vi "ZK Create MB.vi"() -> ()   [LabVIEW 2016, in "质控单元V4.lvlib"]
uses:
  <vilib>/Plasmionique/MB Master/MB_Master_Serial/MB_Master_Serial.lvclass
  C:/Program Files (x86)/National Instruments/LabVIEW 2016/vi.lib/Plasmionique/MB Master/MB_Master/MB_Master.lvclass
  <vilib>/Plasmionique/MB Master/MB_Master_TCP/MB_Master_TCP.lvclass
  <vilib>/Plasmionique/MB Master/MB_Master/MB_Master.lvclass
panel:
  out "auto connected":bool=TRUE
  out "error out":errorcluster
  out "Connected":bool
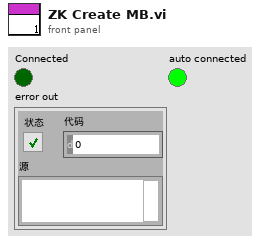
[diagram p1: front panel]
types:
  T1 = cluster{"baud rate (bps)":u32, "stop bits":u16, "parity":u16, "flow control":u16, "timeout":u32, "retries":i32}
  T2 = typedef "质控单元V4.lvlib/质控slave id.ctl" = enum16{"null", "氨氮", "总磷", "总氮", "CODMn", "CODCr"}
  T3 = cluster{"氨氮":bool, "总磷":bool, "总氮":bool, "CODMn":bool, "CODCr":bool, "氨氮总磷":bool, "总磷总氮":bool}
  T4 = typedef "质控单元V4.lvlib/质控仪器状态显示.ctl" = cluster{"运行模式":string, "运行状态":string, "液位状态":string, "告警状态":string, "当前流程":string, "当前步骤":string, "剩余时间":string}
  T5 = typedef "质控单元V4.lvlib/质控仪器状态.ctl" = cluster{"运行状态":enum16{"待机", "润洗", "进样", "定量", "加标", "等待取样", "排液", "异常停机"}, "液位状态":enum16{"无感应", "有感应"}, "告警状态":enum16{"无告警", "液位故障告警", "注射泵异常"}, "当前步骤数":u16, "当前步骤剩余时间":u16, "当前步骤具体操作":enum16{"加标", "进样", "排液", "搅拌", "定量"}, "当前流程":enum16{"待机", "进样流程", "加标流程", "排液流程", "水样润洗流程", "加标润洗流程"}}
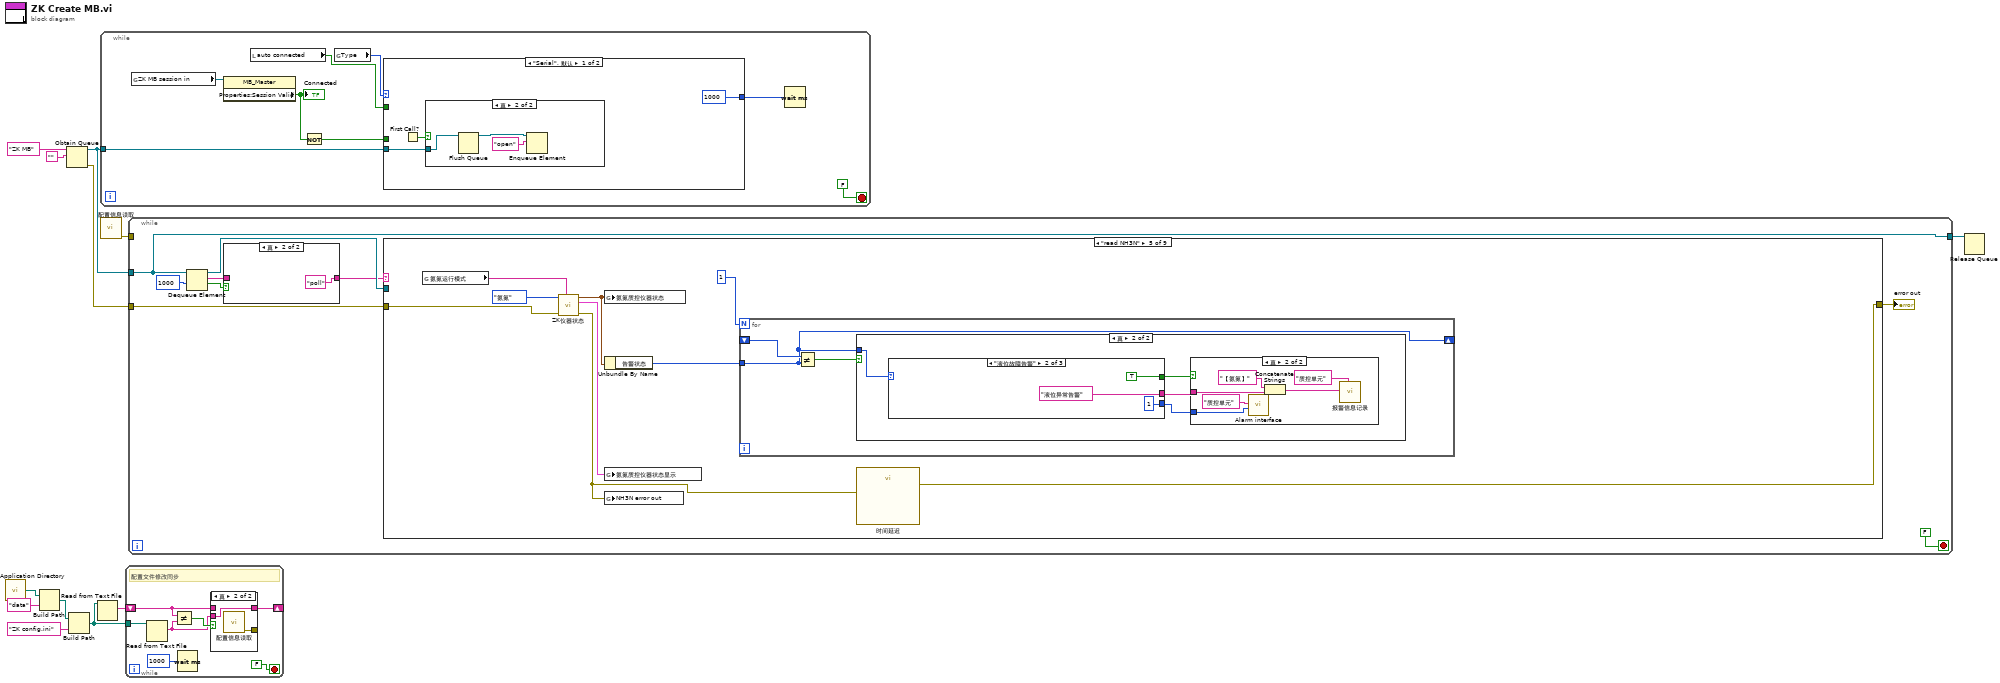
[diagram p0: block diagram]
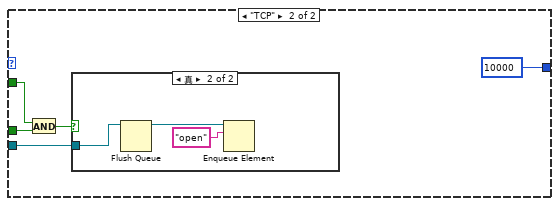
[diagram p4: hidden frame]
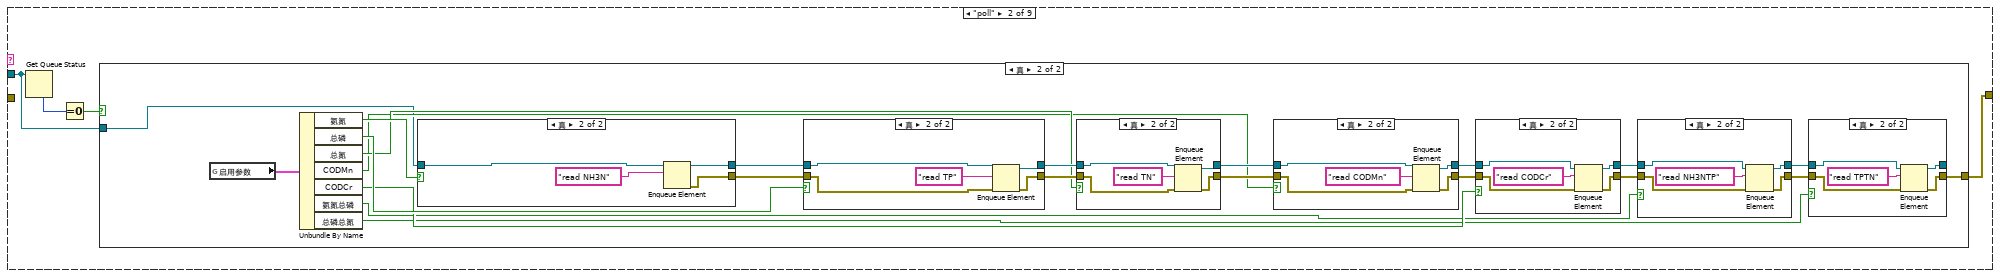
[diagram p8: hidden frame]
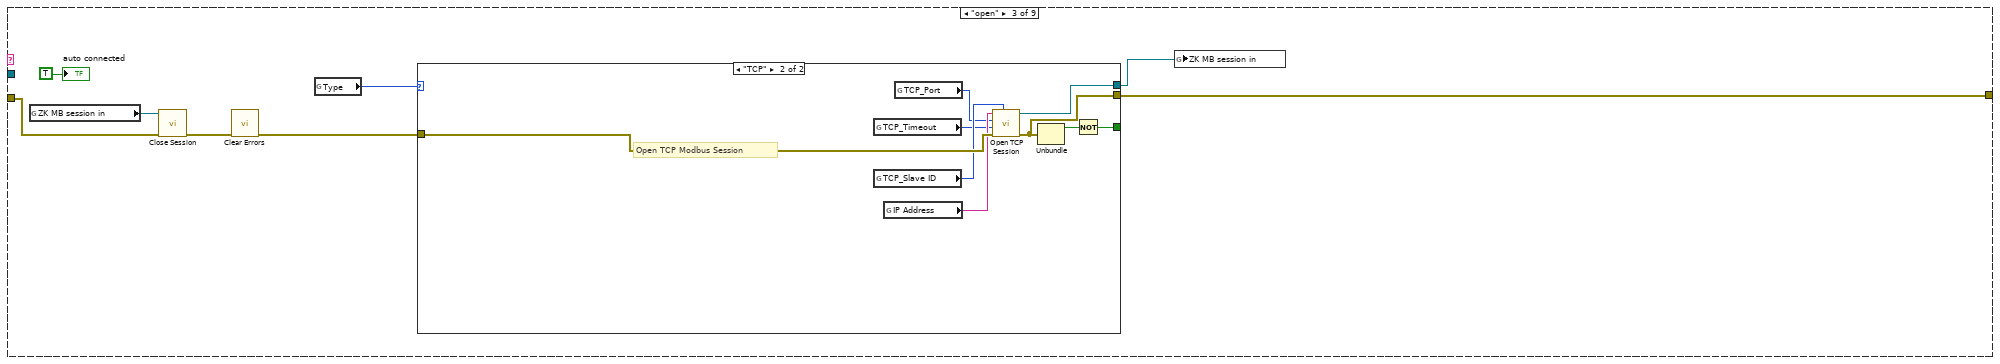
[diagram p17: hidden frame]
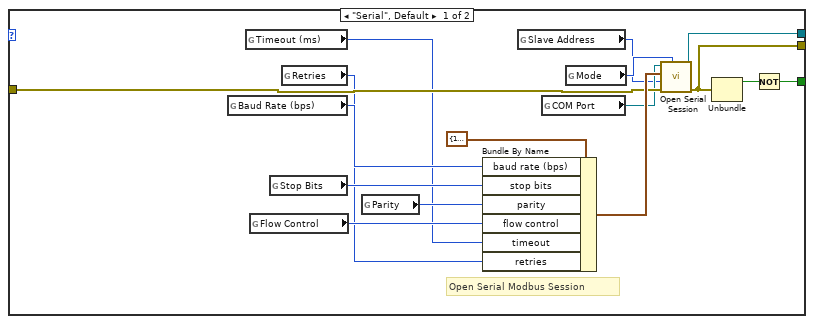
[diagram p18: hidden frame]
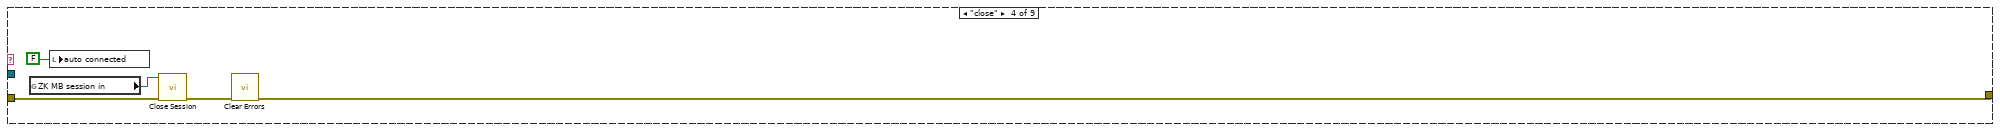
[diagram p19: hidden frame]
diagram:
  n1 = call <vilib>:"Application Directory.vi"() -> ("Application Directory"=w6:path)
  n2 = Build Path(base path=w6, name or relative path="data" ("名称或相对路径")) -> (appended path=w3:path)
  n3 = Obtain Queue(name (unnamed)="ZK MB" ("名称（未命名）"), element data type="") -> (queue out=w10:refnum<queue>, error out=w8:errorcluster)  [unwired: 3 in, 1 out]
  n4 = Build Path(base path=w3, name or relative path="ZK config.ini" ("名称或相对路径")) -> (appended path=w1:path)
  n5 = Read from Text File(file (use dialog)=w1) -> (text=w2:string)  [unwired: 3 in, 3 out]
  n6 = while {
    tunnel: w10 -> [w19]
    stop <- FALSE stop-if-true
    n7 = global read "ZK非断电保存全局变量.vi" "ZK MB session in"() -> (w16:refnum<class "MB_Master.lvclass">)
    n8 = property class="MB_Master"(reference=w16) -> ("Properties:Session Valid"=w15:bool)  [unwired: 1 in, 2 out]
    "Connected" <- w15
    n9 = local read "auto connected"() -> (w14:bool)
    n10 = Not(x=w15) -> (.not. x?=w13:bool)
    n11 = global read "ZK断电保存全局变量.vi" "Type"() -> (w20:enum16{"Serial", "TCP"})
    n12 = case shown="\"Serial\", 默认" w20 {
      tunnel: w19 -> [w23 w31]
      tunnel: [u32 1000 ("等待时间（毫秒）") u32 10000 ("等待时间（毫秒）")] -> w17
      tunnel: w13 -> [_ w29]
      tunnel: w14 -> [_ w27]
      frame "Serial", Default {
        n13 = First Call?() -> (First Call?: T/F=w22:bool)
        n14 = case shown="真" w22 {
          tunnel: w23 -> [_ w26]
          frame False {
          }
          frame True {
            n15 = Flush Queue(queue=w26) -> (queue out=w24:refnum<queue>)  [unwired: 1 in, 2 out]
            n16 = Enqueue Element(queue=w24, element="open") -> ()  [unwired: 2 in, 3 out]
          }
        }
      }
      frame "TCP" {
        n17 = And(x=w27, y=w29) -> (x .and. y?=w28:bool)
        n18 = case shown="真" w28 {
          tunnel: w31 -> [_ w33]
          frame False {
          }
          frame True {
            n19 = Flush Queue(queue=w33) -> (queue out=w32:refnum<queue>)  [unwired: 1 in, 2 out]
            n20 = Enqueue Element(queue=w32, element="open") -> ()  [unwired: 2 in, 3 out]
          }
        }
      }
    }
    n21 = Wait (ms)(milliseconds to wait=w17) -> ()  [unwired: 1 out]
  }
  n22 = call "配置信息读取.vi"() -> ("error out"=w7:errorcluster)  [unwired: 11 in]
  n23 = while {
    shift-right: [w39] -> _
    shift-left: w2 -> [w37]
    tunnel: w1 -> [w41]
    stop <- FALSE stop-if-true
    # "配置文件修改同步"
    n24 = Read from Text File(file (use dialog)=w41) -> (text=w38:string)  [unwired: 3 in, 3 out]
    n25 = Not Equal?(x=w37, y=w38) -> (x != y?=w40:bool)
    n26 = Wait (ms)(milliseconds to wait=u32 1000 ("等待时间（毫秒）")) -> ()  [unwired: 1 out]
    n27 = case shown="真" w40 {
      tunnel: [w42 w44] -> w39
      tunnel: w38 -> [_ w44]
      tunnel: w37 -> [w42 _]
      tunnel: [_ w43] -> _
      frame False {
      }
      frame True {
        n28 = call "配置信息读取.vi"() -> ("error out"=w43:errorcluster)  [unwired: 11 in]
      }
    }
  }
  n29 = while {
    tunnel: w10 -> [w50]
    tunnel: [w50] -> w9
    tunnel: w8 -> [w45]
    tunnel: w7 -> [_]
    stop <- FALSE stop-if-true
    n30 = Dequeue Element(queue=w50, timeout in ms (-1)=1000 ("超时毫秒(-1)")) -> (queue out=w51:refnum<queue>, element=w47:string, timed out?=w48:bool)  [unwired: 1 in, 1 out]
    n31 = case shown="真" w48 {
      tunnel: w47 -> [w54 _]
      tunnel: [w54 "poll"] -> w46
      frame False {
      }
      frame True {
      }
    }
    n32 = case shown="\"read NH3N\"" w46 {
      tunnel: [w56 w60 w132 w165 w173 w201 w229 w257 w285] -> w52
      tunnel: w45 -> [w56 _ w131 w166 w176 w204 w232 w260 w288]
      tunnel: w51 -> [_ w59 _ _ _ _ _ _ _]
      frame Default {
      }
      frame "poll" {
        n33 = Get Queue Status(queue=w59) -> (# elements in queue=w58:i32)  [unwired: 2 in, 7 out]
        n34 = Equal To 0?(x=w58) -> (x = 0?=w57:bool)
        n35 = case shown="真" w57 {
          tunnel: [_ w66] -> w60
          tunnel: w59 -> [_ w61]
          frame False {
          }
          frame True {
            n36 = global read "ZK断电保存全局变量.vi" "启用参数"() -> (w74:T3)
            n37 = Unbundle By Name(w74) -> ("氨氮"=w73:bool, "总磷"=w72:bool, "总氮"=w71:bool, "CODMn"=w65:bool, "CODCr"=w64:bool, "氨氮总磷"=w63:bool, "总磷总氮"=w62:bool)
            n38 = case shown="真" w73 {
              tunnel: w61 -> [w125 w129]
              tunnel: [w125 w128] -> w82
              tunnel: [_ w127] -> w81
              frame False {
              }
              frame True {
                n39 = Enqueue Element(queue=w129, element="read NH3N") -> (queue out=w128:refnum<queue>, error out=w127:errorcluster)  [unwired: 2 in, 1 out]
              }
            }
            n40 = case shown="真" w72 {
              tunnel: w82 -> [w119 w124]
              tunnel: w81 -> [w118 w123]
              tunnel: [w119 w121] -> w80
              tunnel: [w118 w120] -> w77
              frame False {
              }
              frame True {
                n41 = Enqueue Element(queue=w124, element="read TP", error in (no error)=w123) -> (queue out=w121:refnum<queue>, error out=w120:errorcluster)  [unwired: 1 in, 1 out]
              }
            }
            n42 = case shown="真" w71 {
              tunnel: w80 -> [w112 w116]
              tunnel: [w112 w115] -> w70
              tunnel: w77 -> [w111 w114]
              tunnel: [w111 w113] -> w69
              frame False {
              }
              frame True {
                n43 = Enqueue Element(queue=w116, element="read TN", error in (no error)=w114) -> (queue out=w115:refnum<queue>, error out=w113:errorcluster)  [unwired: 1 in, 1 out]
              }
            }
            n44 = case shown="真" w65 {
              tunnel: w70 -> [w91 w95]
              tunnel: [w91 w94] -> w78
              tunnel: w69 -> [w90 w93]
              tunnel: [w90 w92] -> w75
              frame False {
              }
              frame True {
                n45 = Enqueue Element(queue=w95, element="read CODMn", error in (no error)=w93) -> (queue out=w94:refnum<queue>, error out=w92:errorcluster)  [unwired: 1 in, 1 out]
              }
            }
            n46 = case shown="真" w64 {
              tunnel: w78 -> [w84 w89]
              tunnel: w75 -> [w83 w88]
              tunnel: [w83 w86] -> w67
              tunnel: [w84 w85] -> w68
              frame False {
              }
              frame True {
                n47 = Enqueue Element(queue=w89, element="read CODCr", error in (no error)=w88) -> (queue out=w85:refnum<queue>, error out=w86:errorcluster)  [unwired: 1 in, 1 out]
              }
            }
            n48 = case shown="真" w63 {
              tunnel: w68 -> [w105 w109]
              tunnel: [w105 w108] -> w79
              tunnel: w67 -> [w104 w107]
              tunnel: [w104 w106] -> w76
              frame False {
              }
              frame True {
                n49 = Enqueue Element(queue=w109, element="read NH3NTP", error in (no error)=w107) -> (queue out=w108:refnum<queue>, error out=w106:errorcluster)  [unwired: 1 in, 1 out]
              }
            }
            n50 = case shown="真" w62 {
              tunnel: w79 -> [w98 w102]
              tunnel: [w98 w101] -> _
              tunnel: w76 -> [w97 w100]
              tunnel: [w97 w99] -> w66
              frame False {
              }
              frame True {
                n51 = Enqueue Element(queue=w102, element="read TPTN", error in (no error)=w100) -> (queue out=w101:refnum<queue>, error out=w99:errorcluster)  [unwired: 1 in, 1 out]
              }
            }
          }
        }
      }
      frame "open" {
        n52 = global read "ZK非断电保存全局变量.vi" "ZK MB session in"() -> (w134:refnum<class "MB_Master.lvclass">)
        n53 = call-dynamic "Close Session.vi"("error in (no error)"=w131, "MB session in"=w134) -> ("error out"=w136:errorcluster)  [unwired: 9 in]
        n54 = call <vilib>:"Clear Errors.vi"("error in (no error)"=w136) -> ("error out"=w137:errorcluster)  [unwired: 5 in, 1 out]
        n55 = global read "ZK断电保存全局变量.vi" "Type"() -> (w135:enum16{"Serial", "TCP"})
        n56 = case shown="\"TCP\"" w135 {
          tunnel: [w151 w158] -> w133
          tunnel: [w150 w159] -> w132
          tunnel: [w148 w160] -> _
          tunnel: w137 -> [w147 w162]
          frame "Serial", Default {
            # "Open Serial Modbus Session"
            n57 = global read "ZK断电保存全局变量.vi" "Baud Rate (bps)"() -> (w143:u32)
            n58 = global read "ZK断电保存全局变量.vi" "Timeout (ms)"() -> (w139:u32)
            n59 = global read "ZK断电保存全局变量.vi" "Flow Control"() -> (w140:u16)
            n60 = global read "ZK断电保存全局变量.vi" "Stop Bits"() -> (w142:u16)
            n61 = global read "ZK断电保存全局变量.vi" "Retries"() -> (w138:i32)
            n62 = global read "ZK断电保存全局变量.vi" "Parity"() -> (w141:u16)
            n63 = Bundle By Name(cluster=T1 {"baud rate (bps)"=19200, "stop bits"=10, "parity"=0, "flow control"=0, "timeout"=1000, "retries"=1} ("Serial Config"), "baud rate (bps)"=w143, "stop bits"=w142, "parity"=w141, "flow control"=w140, "timeout"=w139, "retries"=w138) -> (w152:T1)
            n64 = global read "ZK断电保存全局变量.vi" "Slave Address"() -> (w144:u8)
            n65 = global read "ZK断电保存全局变量.vi" "COM Port"() -> (w145:refnum<visa-resource-name>)
            n66 = global read "ZK断电保存全局变量.vi" "Mode"() -> (w146:enum16{"RTU", "ASCII"})
            n67 = call <vilib>:"Open Serial Session.vi"("Mode (RTU)"=w146, "Error in"=w147, "Slave ID"=w144, "Serial Config"=w152, "VISA Resource"=w145) -> ("Error out"=w150:errorcluster, "MB_Serial session"=w151:refnum<class "MB_Master_Serial.lvclass">)  [unwired: 5 in]
            n68 = Unbundle(w150) -> ("status"=w149:bool)  [unwired: 2 out]
            n69 = Not(x=w149) -> (.not. x?=w148:bool)
          }
          frame "TCP" {
            # "Open TCP Modbus Session"
            n70 = global read "ZK断电保存全局变量.vi" "TCP_Timeout"() -> (w154:i32)
            n71 = global read "ZK断电保存全局变量.vi" "TCP_Slave ID"() -> (w157:u8)
            n72 = global read "ZK断电保存全局变量.vi" "IP Address"() -> (w156:string)
            n73 = global read "ZK断电保存全局变量.vi" "TCP_Port"() -> (w155:u16)
            n74 = call <vilib>:"Open TCP Session.vi"("Slave ID (255)"=w157, "error in (no error)"=w162, "Timeout (10000)"=w154, "Port (502)"=w155, "IP Address"=w156) -> ("error out"=w159:errorcluster, "MB_TCP session"=w158:refnum<class "MB_Master_TCP.lvclass">)  [unwired: 5 in]
            n75 = Unbundle(w159) -> ("status"=w161:bool)  [unwired: 2 out]
            n76 = Not(x=w161) -> (.not. x?=w160:bool)
          }
        }
        n77 = global write "ZK非断电保存全局变量.vi" "ZK MB session in"(w133) -> ()
        "auto connected" <- TRUE
      }
      frame "close" {
        n78 = global read "ZK非断电保存全局变量.vi" "ZK MB session in"() -> (w164:refnum<class "MB_Master.lvclass">)
        n79 = local write "auto connected"(FALSE ("auto connected")) -> ()
        n80 = call-dynamic "Close Session.vi"("error in (no error)"=w166, "MB session in"=w164) -> ("error out"=w167:errorcluster)  [unwired: 9 in]
        n81 = call <vilib>:"Clear Errors.vi"("error in (no error)"=w167) -> ("error out"=w165:errorcluster)  [unwired: 5 in, 1 out]
      }
      frame "read NH3N" {
        n82 = global read "ZK非断电保存全局变量.vi" "氨氮运行模式"() -> (w168:string)
        n83 = call "ZK仪器状态.vi"("运行模式"=w168, "error in (no error)"=w176, "Slave ID"=质控slave_id."氨氮") -> ("error out"=w174:errorcluster, "质控仪器状态显示"=w172:T4, "质控仪器状态"=w171:T5)  [unwired: 6 in]
        n84 = global write "ZK非断电保存全局变量.vi" "氨氮质控仪器状态"(w171) -> ()
        n85 = Unbundle By Name(w171) -> ("告警状态"=w169:enum16{"无告警", "液位故障告警", "注射泵异常"})
        n86 = global write "ZK非断电保存全局变量.vi" "氨氮质控仪器状态显示"(w172) -> ()
        n87 = global write "ZK非断电保存全局变量.vi" "NH3N error out"(w174) -> ()
        n88 = for {
          N: 1 -> [_]
          shift-right: [w178] -> _
          shift-left: _ -> [w179]
          tunnel: w169 -> [w178]
          n89 = Not Equal?(x=w179, y=w178) -> (x != y?=w177:bool)
          n90 = case shown="真" w177 {
            tunnel: w178 -> [_ w183]
            frame False {
            }
            frame True {
              n91 = case shown="\"液位故障告警\"" w183 {
                tunnel: [_ "液位异常告警" ("字符串") "柱塞泵故障告警" ("字符串")] -> w181
                tunnel: [_ TRUE TRUE] -> w182
                tunnel: [_ 1 ("code") 2 ("code")] -> w180
                frame "无告警", Default {
                }
                frame "液位故障告警" {
                }
                frame "注射泵异常" {
                }
              }
              n92 = case shown="真" w182 {
                tunnel: w181 -> [_ w194]
                tunnel: w180 -> [_ w190]
                frame False {
                }
                frame True {
                  n93 = call "Alarm interface.vi"("code"=w190, "模块名称"="质控单元") -> ()  [unwired: 9 in, 1 out]
                  n94 = Concatenate Strings("【氨氮】" ("字符串"), w194) -> (w192:string)
                  n95 = call "报警信息记录.vi"("参数"="质控单元", "报警信息"=w192) -> ()  [unwired: 9 in, 1 out]
                }
              }
            }
          }
        }
        n96 = call "时间延迟"("error in (no error)"=w174) -> ("error out"=w173:errorcluster)  [unwired: 10 in]
      }
      frame "read TP" {
        n97 = global read "ZK非断电保存全局变量.vi" "总磷运行模式"() -> (w196:string)
        n98 = call "ZK仪器状态.vi"("运行模式"=w196, "error in (no error)"=w204, "Slave ID"=质控slave_id."总磷") -> ("error out"=w202:errorcluster, "质控仪器状态显示"=w200:T4, "质控仪器状态"=w199:T5)  [unwired: 6 in]
        n99 = global write "ZK非断电保存全局变量.vi" "总磷质控仪器状态"(w199) -> ()
        n100 = Unbundle By Name(w199) -> ("告警状态"=w198:enum16{"无告警", "液位故障告警", "注射泵异常"})
        n101 = global write "ZK非断电保存全局变量.vi" "总磷质控仪器状态显示"(w200) -> ()
        n102 = global write "ZK非断电保存全局变量.vi" "tp error out"(w202) -> ()
        n103 = for {
          N: 1 -> [_]
          shift-right: [w206] -> _
          shift-left: _ -> [w207]
          tunnel: w198 -> [w206]
          n104 = Not Equal?(x=w207, y=w206) -> (x != y?=w205:bool)
          n105 = case shown="真" w205 {
            tunnel: w206 -> [_ w211]
            frame False {
            }
            frame True {
              n106 = case shown="\"液位故障告警\"" w211 {
                tunnel: [_ "液位异常告警" ("字符串") "柱塞泵故障告警" ("字符串")] -> w209
                tunnel: [_ TRUE TRUE] -> w210
                tunnel: [_ 1 ("code") 2 ("code")] -> w208
                frame "无告警", Default {
                }
                frame "液位故障告警" {
                }
                frame "注射泵异常" {
                }
              }
              n107 = case shown="真" w210 {
                tunnel: w209 -> [_ w222]
                tunnel: w208 -> [_ w218]
                frame False {
                }
                frame True {
                  n108 = call "Alarm interface.vi"("code"=w218, "模块名称"="质控单元") -> ()  [unwired: 9 in, 1 out]
                  n109 = Concatenate Strings("【总磷】" ("字符串"), w222) -> (w220:string)
                  n110 = call "报警信息记录.vi"("参数"="质控单元", "报警信息"=w220) -> ()  [unwired: 9 in, 1 out]
                }
              }
            }
          }
        }
        n111 = call "时间延迟2"("error in (no error)"=w202) -> ("error out"=w201:errorcluster)  [unwired: 10 in]
      }
      frame "read TN" {
        n112 = global read "ZK非断电保存全局变量.vi" "总氮运行模式"() -> (w224:string)
        n113 = call "ZK仪器状态.vi"("运行模式"=w224, "error in (no error)"=w232, "Slave ID"=质控slave_id."总氮") -> ("error out"=w230:errorcluster, "质控仪器状态显示"=w228:T4, "质控仪器状态"=w227:T5)  [unwired: 6 in]
        n114 = global write "ZK非断电保存全局变量.vi" "总氮质控仪器状态"(w227) -> ()
        n115 = Unbundle By Name(w227) -> ("告警状态"=w226:enum16{"无告警", "液位故障告警", "注射泵异常"})
        n116 = global write "ZK非断电保存全局变量.vi" "总氮质控仪器状态显示"(w228) -> ()
        n117 = global write "ZK非断电保存全局变量.vi" "tn error out"(w230) -> ()
        n118 = for {
          N: 1 -> [_]
          shift-right: [w234] -> _
          shift-left: _ -> [w235]
          tunnel: w226 -> [w234]
          n119 = Not Equal?(x=w235, y=w234) -> (x != y?=w233:bool)
          n120 = case shown="真" w233 {
            tunnel: w234 -> [_ w239]
            frame False {
            }
            frame True {
              n121 = case shown="\"液位故障告警\"" w239 {
                tunnel: [_ "液位异常告警" ("字符串") "柱塞泵故障告警" ("字符串")] -> w237
                tunnel: [_ TRUE TRUE] -> w238
                tunnel: [_ 1 ("code") 2 ("code")] -> w236
                frame "无告警", Default {
                }
                frame "液位故障告警" {
                }
                frame "注射泵异常" {
                }
              }
              n122 = case shown="真" w238 {
                tunnel: w237 -> [_ w250]
                tunnel: w236 -> [_ w246]
                frame False {
                }
                frame True {
                  n123 = Concatenate Strings("【总氮】" ("字符串"), w250) -> (w248:string)
                  n124 = call "Alarm interface.vi"("code"=w246, "模块名称"="质控单元") -> ()  [unwired: 9 in, 1 out]
                  n125 = call "报警信息记录.vi"("参数"="质控单元", "报警信息"=w248) -> ()  [unwired: 9 in, 1 out]
                }
              }
            }
          }
        }
        n126 = call "时间延迟3"("error in (no error)"=w230) -> ("error out"=w229:errorcluster)  [unwired: 10 in]
      }
      frame "read CODMn" {
        n127 = global read "ZK非断电保存全局变量.vi" "CODMn运行模式"() -> (w252:string)
        n128 = call "ZK仪器状态.vi"("运行模式"=w252, "error in (no error)"=w260, "Slave ID"=质控slave_id."CODMn") -> ("error out"=w258:errorcluster, "质控仪器状态显示"=w256:T4, "质控仪器状态"=w255:T5)  [unwired: 6 in]
        n129 = global write "ZK非断电保存全局变量.vi" "CODMn质控仪器状态"(w255) -> ()
        n130 = Unbundle By Name(w255) -> ("告警状态"=w254:enum16{"无告警", "液位故障告警", "注射泵异常"})
        n131 = global write "ZK非断电保存全局变量.vi" "CODMn质控仪器状态显示"(w256) -> ()
        n132 = global write "ZK非断电保存全局变量.vi" "CODMn error out"(w258) -> ()
        n133 = for {
          N: 1 -> [_]
          shift-right: [w262] -> _
          shift-left: _ -> [w263]
          tunnel: w254 -> [w262]
          n134 = Not Equal?(x=w263, y=w262) -> (x != y?=w261:bool)
          n135 = case shown="真" w261 {
            tunnel: w262 -> [_ w267]
            frame False {
            }
            frame True {
              n136 = case shown="\"无告警\", 默认" w267 {
                tunnel: [_ "液位异常告警" ("字符串") "柱塞泵故障告警" ("字符串")] -> w265
                tunnel: [_ TRUE TRUE] -> w266
                tunnel: [_ 1 ("code") 2 ("code")] -> w264
                frame "无告警", Default {
                }
                frame "液位故障告警" {
                }
                frame "注射泵异常" {
                }
              }
              n137 = case shown="真" w266 {
                tunnel: w265 -> [_ w278]
                tunnel: w264 -> [_ w274]
                frame False {
                }
                frame True {
                  n138 = call "Alarm interface.vi"("code"=w274, "模块名称"="质控单元") -> ()  [unwired: 9 in, 1 out]
                  n139 = Concatenate Strings("【CODMn】" ("字符串"), w278) -> (w276:string)
                  n140 = call "报警信息记录.vi"("参数"="质控单元", "报警信息"=w276) -> ()  [unwired: 9 in, 1 out]
                }
              }
            }
          }
        }
        n141 = call "时间延迟4"("error in (no error)"=w258) -> ("error out"=w257:errorcluster)  [unwired: 10 in]
      }
      frame "read CODCr" {
        n142 = global read "ZK非断电保存全局变量.vi" "CODCr运行模式"() -> (w280:string)
        n143 = call "ZK仪器状态.vi"("运行模式"=w280, "error in (no error)"=w288, "Slave ID"=质控slave_id."CODCr") -> ("error out"=w286:errorcluster, "质控仪器状态显示"=w284:T4, "质控仪器状态"=w283:T5)  [unwired: 6 in]
        n144 = global write "ZK非断电保存全局变量.vi" "CODCr质控仪器状态"(w283) -> ()
        n145 = Unbundle By Name(w283) -> ("告警状态"=w282:enum16{"无告警", "液位故障告警", "注射泵异常"})
        n146 = global write "ZK非断电保存全局变量.vi" "CODcr质控仪器状态显示"(w284) -> ()
        n147 = global write "ZK非断电保存全局变量.vi" "CODCr error out"(w286) -> ()
        n148 = for {
          N: 1 -> [_]
          shift-right: [w290] -> _
          shift-left: _ -> [w291]
          tunnel: w282 -> [w290]
          n149 = Not Equal?(x=w291, y=w290) -> (x != y?=w289:bool)
          n150 = case shown="真" w289 {
            tunnel: w290 -> [_ w295]
            frame False {
            }
            frame True {
              n151 = case shown="\"注射泵异常\"" w295 {
                tunnel: [_ "液位异常告警" ("字符串") "柱塞泵故障告警" ("字符串")] -> w294
                tunnel: [_ TRUE TRUE] -> w293
                tunnel: [_ 1 ("元素") 2 ("元素")] -> w292
                frame "无告警", Default {
                }
                frame "液位故障告警" {
                }
                frame "注射泵异常" {
                }
              }
              n152 = case shown="真" w293 {
                tunnel: w294 -> [_ w300]
                tunnel: w292 -> [_ w296]
                frame False {
                }
                frame True {
                  n153 = Concatenate Strings("【CODCr】" ("字符串"), w300) -> (w298:string)
                  n154 = call "Alarm interface.vi"("code"=w296, "模块名称"="质控单元") -> ()  [unwired: 9 in, 1 out]
                  n155 = call "报警信息记录.vi"("参数"="质控单元", "报警信息"=w298) -> ()  [unwired: 9 in, 1 out]
                }
              }
            }
          }
        }
        n156 = call "时间延迟5"("error in (no error)"=w286) -> ("error out"=w285:errorcluster)  [unwired: 10 in]
      }
    }
    "error out" <- w52
  }
  n157 = Release Queue(queue=w9) -> ()  [unwired: 2 in, 3 out]
